vi "Fetch Rooms List and Size Limits.vi"(0 "Rooms Manager Model in":refnum<class "Rooms Manager Model.lvclass">, 5 "Room Size":string, 11 "error in (no error)":errorcluster) -> (4 "Rooms Manager Model out":refnum<class "Rooms Manager Model.lvclass">, 15 "error out":errorcluster)   [LabVIEW 2023, in "Rooms Manager Model.lvlib" / "Rooms Manager Model.lvclass"]
uses:
  Rooms Manager Model.lvclass
  Rooms Manager Model.lvclass/Rooms Manager Model.ctl
  Guest Manager Model/Guest Manager Model Messages/Update Rooms List Msg/Update Rooms List Msg.lvclass/Update Rooms List Msg.ctl
  <vilib>/ActorFramework/Message Enqueuer/Message Enqueuer.lvclass/Message Enqueuer.ctl
  Guest Manager Model/Guest Manager Model Messages/Update Size Limits Msg/Update Size Limits Msg.lvclass/Update Size Limits Msg.ctl
  <vilib>/ActorFramework/Message Enqueuer/Enqueue.vi
  Guest Manager Model/Guest Manager Model Messages/Update Rooms List Msg/Update Rooms List Msg.lvclass
  Guest Manager Model/Guest Manager Model Messages/Update Size Limits Msg/Update Size Limits Msg.lvclass
  <vilib>/ActorFramework/Message Priority Queue/Priority Enqueue.vi
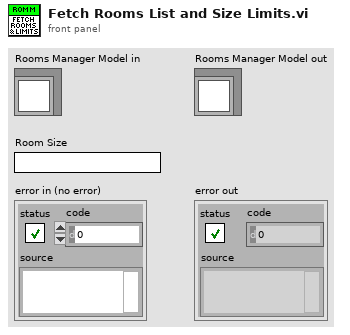
[diagram p1: front panel]
types:
  T1 = typedef "Central Data Manager.lvlib/Central Data Manager.lvclass/Room Size Details.ctl" = cluster{"Size":string, "Cost Per Day (Rs)":u32, "Occupancy Limit (Adult)":u32, "Occupancy Limit (Children)":u32}
  T2 = typedef "Central Data Manager.lvlib/Central Data Manager.lvclass/Room Details.ctl" = cluster{"Room No":string, "Room Size":string, "Room Occupancy Status":T3, "Guest Details":T4, "Occupancy Count (Adult)":u32, "Occupancy Count (Children)":u32, "Check-in Time":timestamp, "Check-out Time":timestamp}
  T3 = typedef "Central Data Manager.lvlib/Central Data Manager.lvclass/Room Occupancy Status.ctl" = enum16{"Not Occupied", "Occupied", "Under Maintainance", "Not Servicable"}
  T4 = typedef "Central Data Manager.lvlib/Central Data Manager.lvclass/Guest Details.ctl" = cluster{"Contact Number":string, "Primary Guest Name":string}
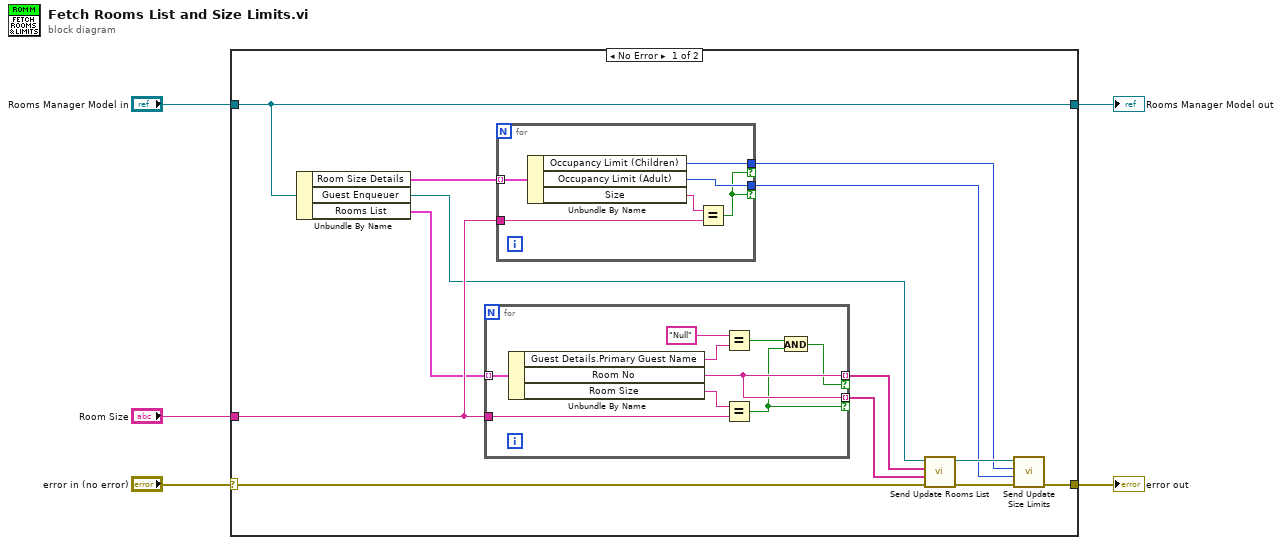
[diagram p0: block diagram]
diagram:
  n1 = case shown="No Error" "error in (no error)" {
    selector: "error in (no error)" -> [w17 w34]
    tunnel: [w15 w34] -> w2
    tunnel: "Rooms Manager Model in" -> [w11 w35]
    tunnel: [w11 w35] -> w3
    tunnel: "Room Size" -> [w10 _]
    frame No Error {
      n2 = Unbundle By Name(w11) -> ("Room Size Details"=w18:T1[], "Guest Enqueuer"=w7:refnum<class "Message Enqueuer.lvclass">, "Rooms List"=w6:T2[])
      n3 = for {
        tunnel: w6 -> [w33] mode=indexing
        tunnel: w10 -> [w31]
        tunnel: [w30] -> w8 mode=indexing if=w29
        tunnel: [w30] -> w9 mode=indexing if=w28
        n4 = Unbundle By Name(w33) -> ("Guest Details.Primary Guest Name"=w27:string, "Room No"=w30:string, "Room Size"=w32:string)
        n5 = Equal?(x="Null", y=w27) -> (x = y?=w25:bool)
        n6 = Equal?(x=w32, y=w31) -> (x = y?=w28:bool)
        n7 = And(x=w25, y=w28) -> (x .and. y?=w29:bool)
      }
      n8 = for {
        tunnel: w18 -> [w24] mode=indexing
        tunnel: w10 -> [w20]
        tunnel: [w23] -> w13 if=w19
        tunnel: [w22] -> w12 if=w19
        n9 = Unbundle By Name(w24) -> ("Occupancy Limit (Children)"=w23:u32, "Occupancy Limit (Adult)"=w22:u32, "Size"=w21:string)
        n10 = Equal?(x=w21, y=w20) -> (x = y?=w19:bool)
      }
      n11 = call "Send Update Rooms List.vi"("error in (no error)"=w17, "All Rooms"=w9, "Available Rooms"=w8, "Message Enqueuer"=w7) -> ("error out"=w16:errorcluster, "Message Enqueuer out"=w14:refnum<class "Message Enqueuer.lvclass">)  [unwired: 6 in]
      n12 = call "Send Update Size Limits.vi"("error in (no error)"=w16, "Adult Count"=w12, "Children Count"=w13, "Message Enqueuer"=w14) -> ("error out"=w15:errorcluster)  [unwired: 6 in, 1 out]
    }
    frame Error {
    }
  }
  "error out" <- w2
  "Rooms Manager Model out" <- w3
